vi "fpgatrig.vi"(0 "Distance detected":fxp<+/-,64,32>, 5 "sensor angle (Radiens)":fxp<+/-,64,32>, 7 "stop":bool, 9 "Sensor position y":fxp<+/-,64,32>, 11 "Sensor position x":fxp<+/-,64,32>) -> (4 "Detected x Cord":fxp<+/-,64,32>, 6 "Detected y Cord":fxp<+/-,64,32>)   [LabVIEW 2012]
uses:
  <vilib>/rvi/FXPMathLib/FxpSinAndCos/subVIs/nifxpmath_SinAndCos_SimConfig.ctl
  <vilib>/rvi/FXPMathLib/FxpSinAndCos/simVIs/DllFxpSinAndCosTemp_sub.vi
  <vilib>/rvi/FXPMathLib/FxpSinAndCos/XNode/nifxpmath_SinAndCos.xnode
  <vilib>/rvi/FXPMathLib/FxpMul/XNode/nifxpmath_Multiplier.xnode
  <vilib>/rvi/FXPMathLib/FxpAdd/XNode/nifxpmath_Add.xnode
  <vilib>/rvi/FXPMathLib/sim/FxpSim.dll
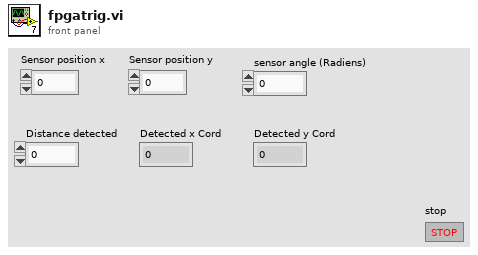
[diagram p1: front panel]
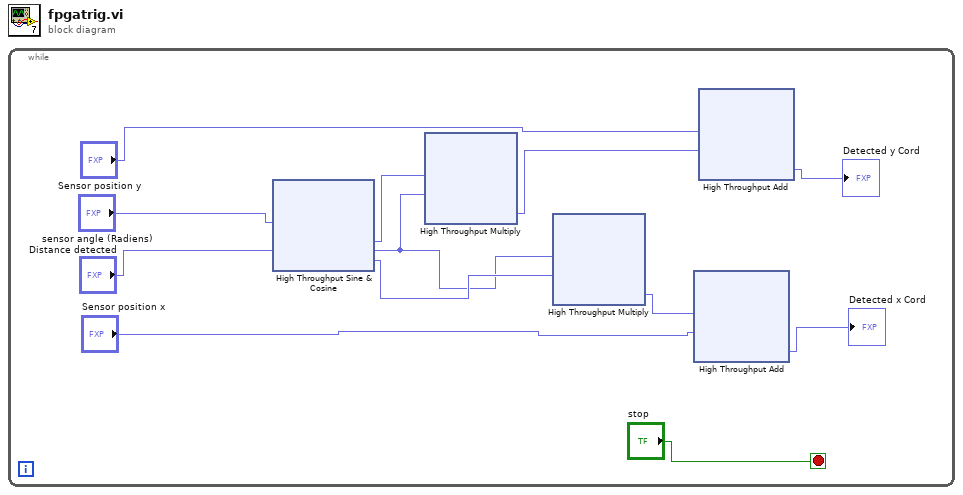
[diagram p0: block diagram]
diagram:
  n1 = while {
    stop <- "stop" stop-if-true
    n2 = xnode "High Throughput Sine & Cosine"("x (pi)"="sensor angle (Radiens)") -> ("sin(x)"=w5:fxp<+/-,16,2>, "cos(x)"=w9:fxp<+/-,16,2>)
    n3 = xnode "High Throughput Multiply"("x"=w5, "y"="Distance detected") -> ("x*y"=w3:fxp<+/-,64,34>)
    n4 = xnode "High Throughput Multiply"("x"="Distance detected", "y"=w9) -> ("x*y"=w7:fxp<+/-,64,34>)
    n5 = xnode "High Throughput Add"("x"=w7, "y"="Sensor position x") -> ("x+y"=→"Detected x Cord":fxp<+/-,64,35>)
    n6 = xnode "High Throughput Add"("x"="Sensor position y", "y"=w3) -> ("x+y"=→"Detected y Cord":fxp<+/-,64,35>)
  }
